vi "RandomizeTargetSet.vi"(1 "Target set":i16[](array[ring]) items=["1", "2", "3", "4"]) -> (0 "Target set rand order":i16[](array[ring]) items=["1", "2", "3", "4"])   [LabVIEW 2010]
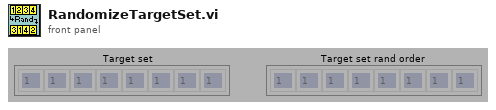
[diagram p1: front panel]
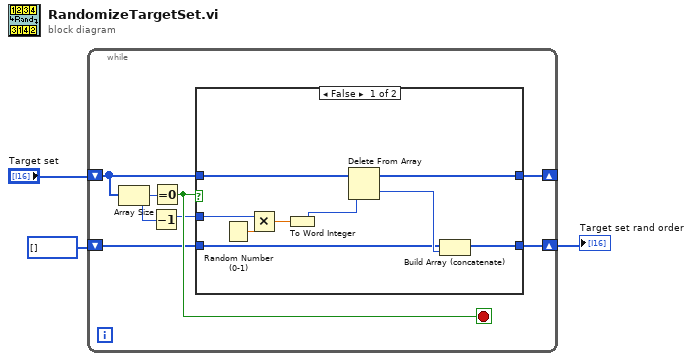
[diagram p0: block diagram]
diagram:
  n1 = while {
    shift-right: [w7] -> _
    shift-left: "Target set" -> [w8]
    shift-right: [w5] -> w1
    shift-left: i16[] [] -> [w4]
    stop <- w10 stop-if-true
    n2 = Array Size(array=w8) -> (size(s)=w9:i32)
    n3 = Decrement(x=w9) -> (x-1=w6:i32)
    n4 = Equal To 0?(x=w9) -> (x = 0?=w10:bool)
    n5 = case shown="False" w10 {
      tunnel: w6 -> [w18 _]
      tunnel: w8 -> [w16 w21]
      tunnel: [w14 w21] -> w7
      tunnel: [w12 w20] -> w5
      tunnel: w4 -> [w11 w20]
      frame False {
        n6 = Random Number (0-1)() -> (number: 0 to 1=w19:dbl)
        n7 = Multiply(x=w18, y=w19) -> (x*y=w17:dbl)
        n8 = To Word Integer(number=w17) -> (16bit integer=w15:i16)
        n9 = Delete From Array(array=w16, index=w15) -> (deleted portion=w13:i16, array with subset deleted=w14:i16[])  [unwired: 1 in]
        n10 = Build Array (concatenate)(w11, w13) -> (w12:i16[])
      }
      frame True {
      }
    }
  }
  "Target set rand order" <- w1
